vi "-Move Poly-.vi"   [LabVIEW 2010, in "4150 ringbot v1.lvrbt"]
uses:
  4150 ringbot v1.lvrbt
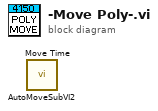
[diagram p0: block diagram]
diagram:
  n1 = call "AutoMoveSubVI2.vi"() -> ()  [unwired: 12 in]
  n2 = call "Move Time.vi"() -> ()  [unwired: 15 in, 1 out]
